vi "Test_波形显示.vi"(3 "error in (no error)":errorcluster, 4 "通道名输入":string[](array[string])=["行程"], 5 "文件路径":path=path "C:/Users/Xiang MU/Desktop/实验文件夹/DR96-03-5/SV1/SV1-开启关闭.tdms") -> (0 "error out":errorcluster, 2 "波形图":waveform(dbl)[](graph))   [LabVIEW 2013]
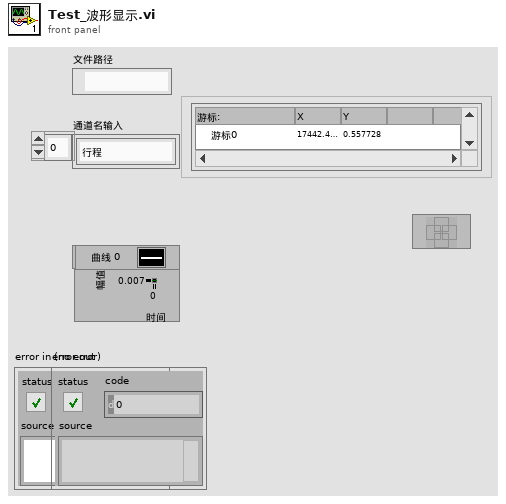
[diagram p1: front panel]
types:
  T1 = enum16{"open", "open or create", "create or replace", "create", "open (read-only)"}
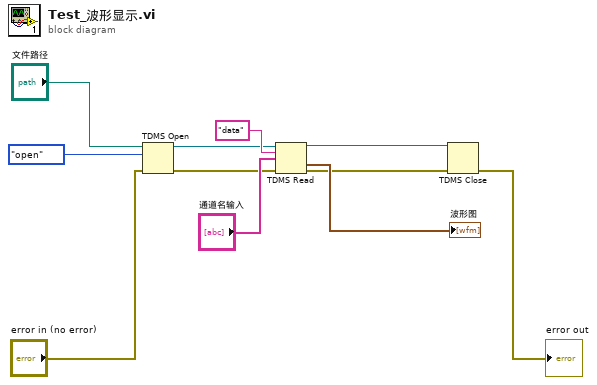
[diagram p0: block diagram]
diagram:
  n1 = TDMS Open(8:"error in (no error)", 10:T1."open" ("操作(0:open)"), 11:"文件路径") -> (0:w3:errorcluster, 3:w6:refnum<k34>)  [unwired: 4 in]
  n2 = TDMS Read(0:w6, 5:"data" ("组名称输入"), 7:"通道名输入", 11:w3) -> (4:w5:refnum<k34>, 10:→"波形图":waveform(dbl)[], 15:w2:errorcluster)  [unwired: 4 in, 3 out]
  n3 = TDMS Close(8:w2, 11:w5) -> (0:→"error out":errorcluster)  [unwired: 1 out]
